vi "Async Thread.vi"(11 "TCP网络连接引用句柄":refnum<k5>) -> ()   [LabVIEW 2019, in "HTTP Server.lvlib"]
uses:
  HTTP Server.lvlib
  Async Thread.ctl
panel:
  out "路径":path
  in  "停止":bool
  out "添加的路径":path
  out "error out":errorcluster caption="错误输出"
  in  "error in (no error)":errorcluster caption="错误输入（无错误）"
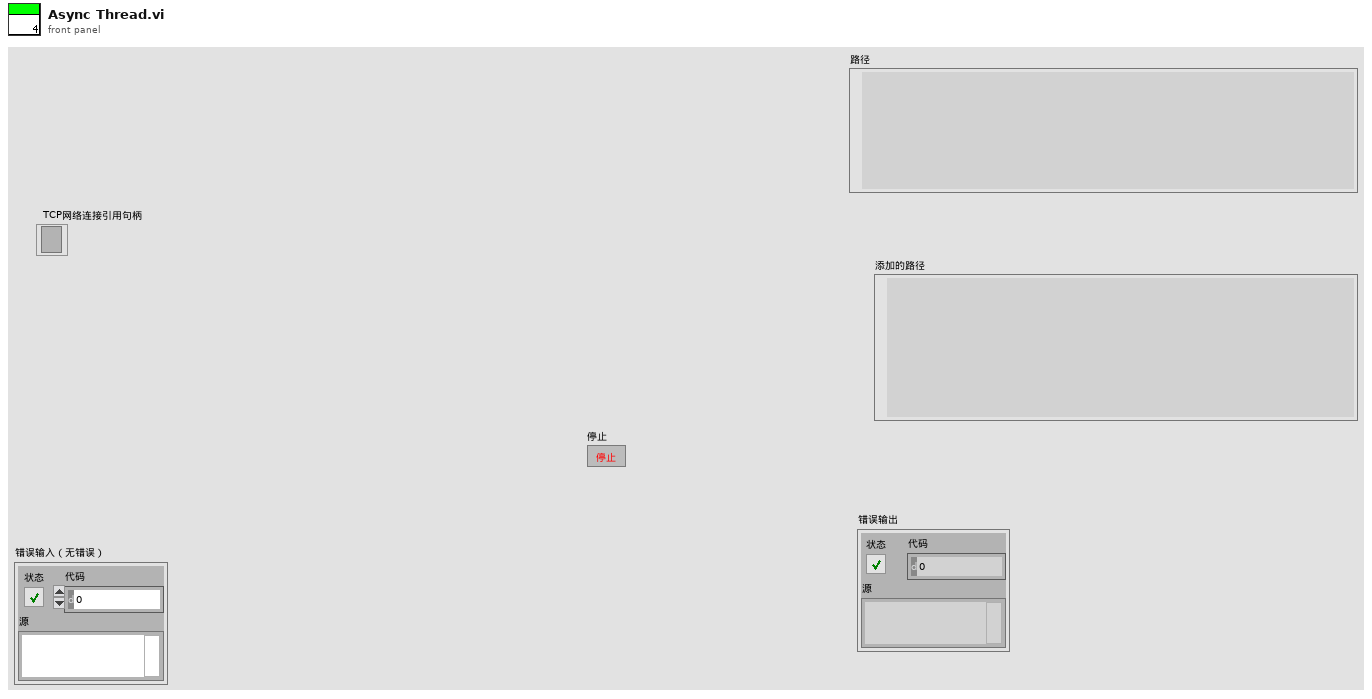
[diagram p1: front panel]
types:
  T1 = typedef "HTTP Server.lvlib/Async Thread.ctl" = cluster{"HTTP报文":string, "请求报文首部":cluster{"请求行":cluster{"方法":string, "URI":string, "表单数据":cluster{"key":string[], "value":string[]}, "HTTP版本":string}, "首部字段":cluster{"key":string[], "value":string[]}}, "请求报文主体":string, "响应报文主体":string, "响应代码":u16, "响应报文首部":string, "Redis TCP引用":refnum<k5>}
  T2 = enum32{"invalid app kind", "Development System", "Run Time System", "Student Edition", "Embedded LabVIEW", "Evaluation", "Custom"}
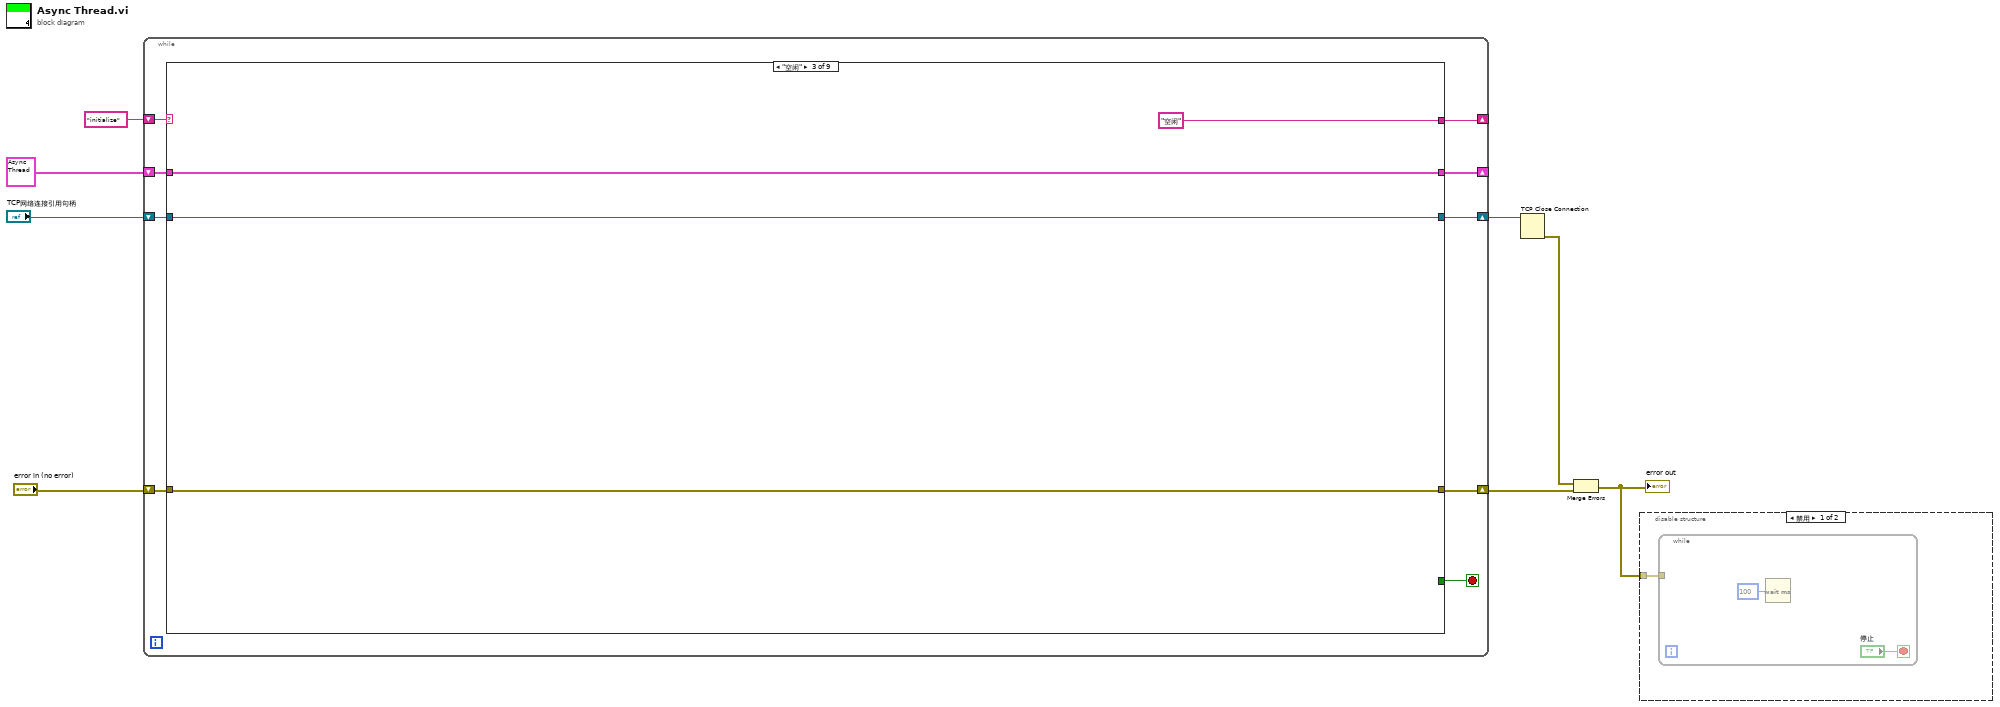
[diagram p0: block diagram]
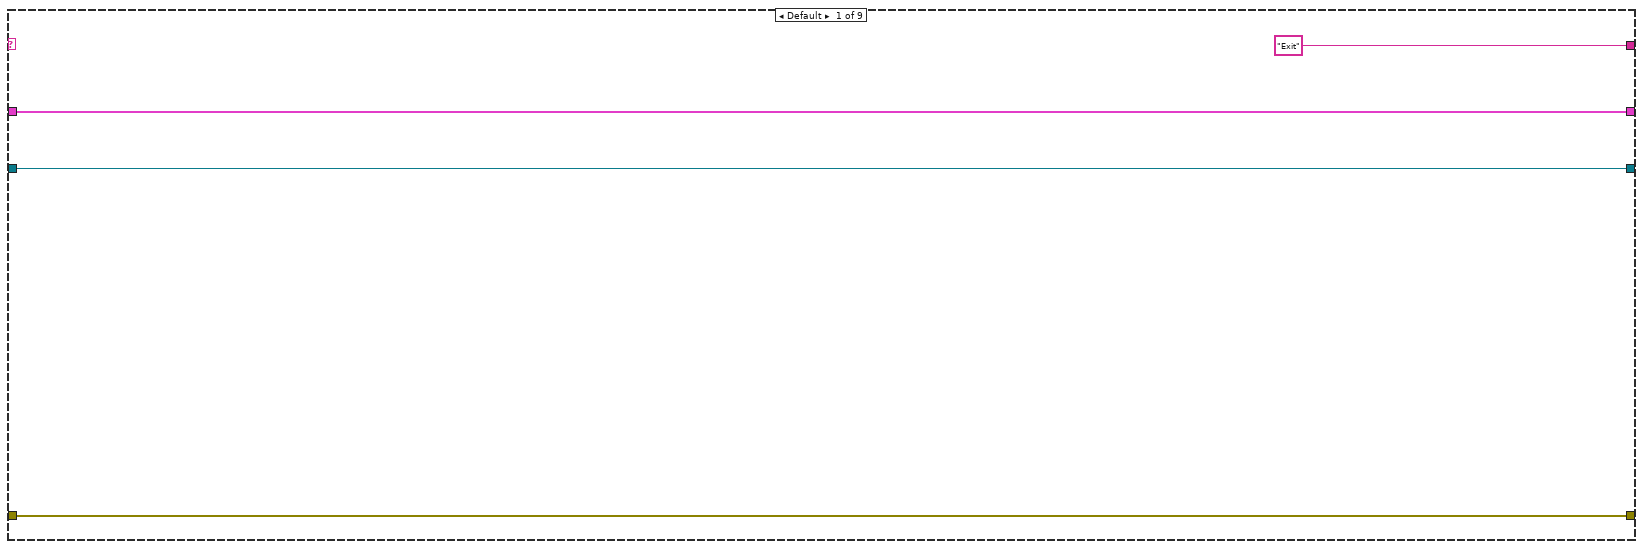
[diagram p3: hidden frame]
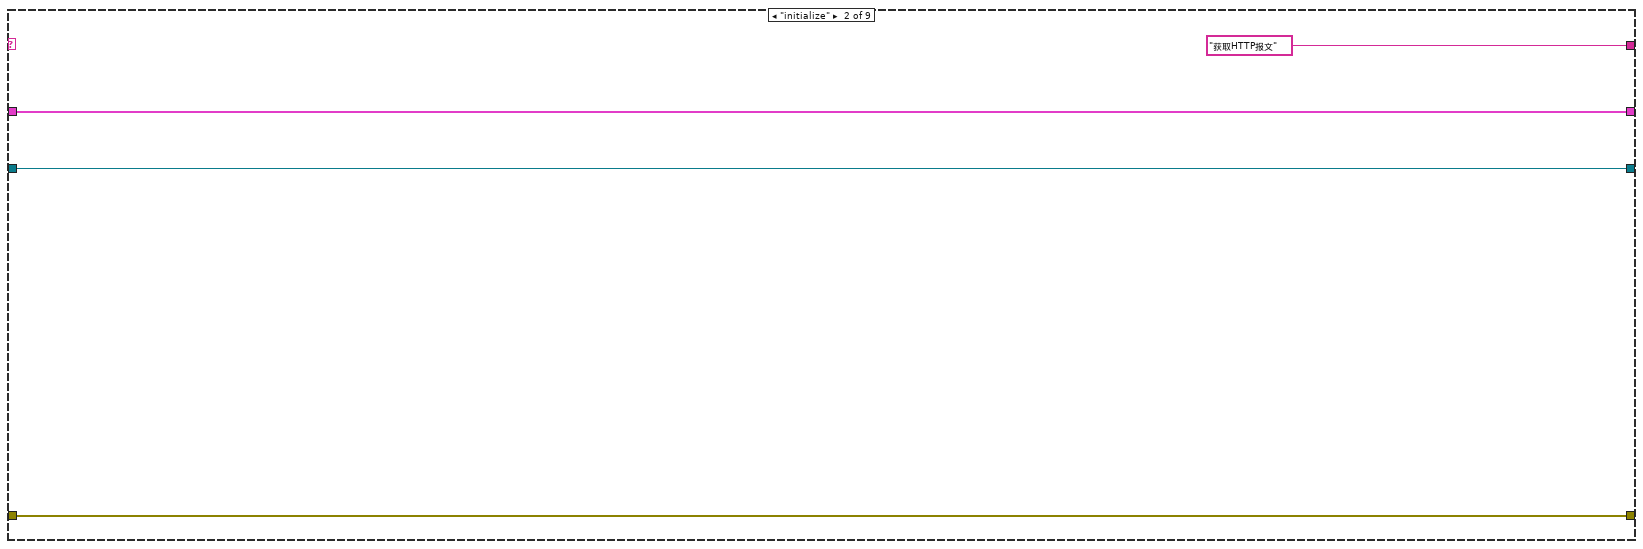
[diagram p4: hidden frame]
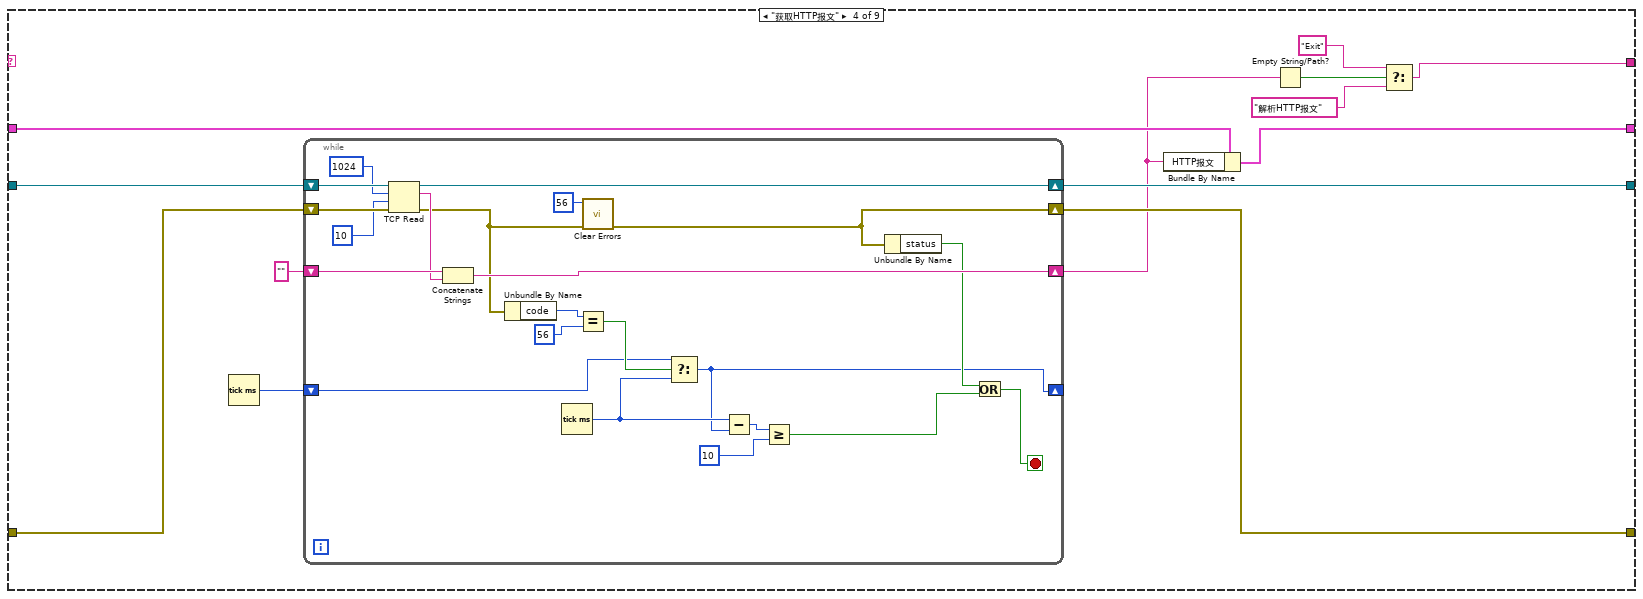
[diagram p5: hidden frame]
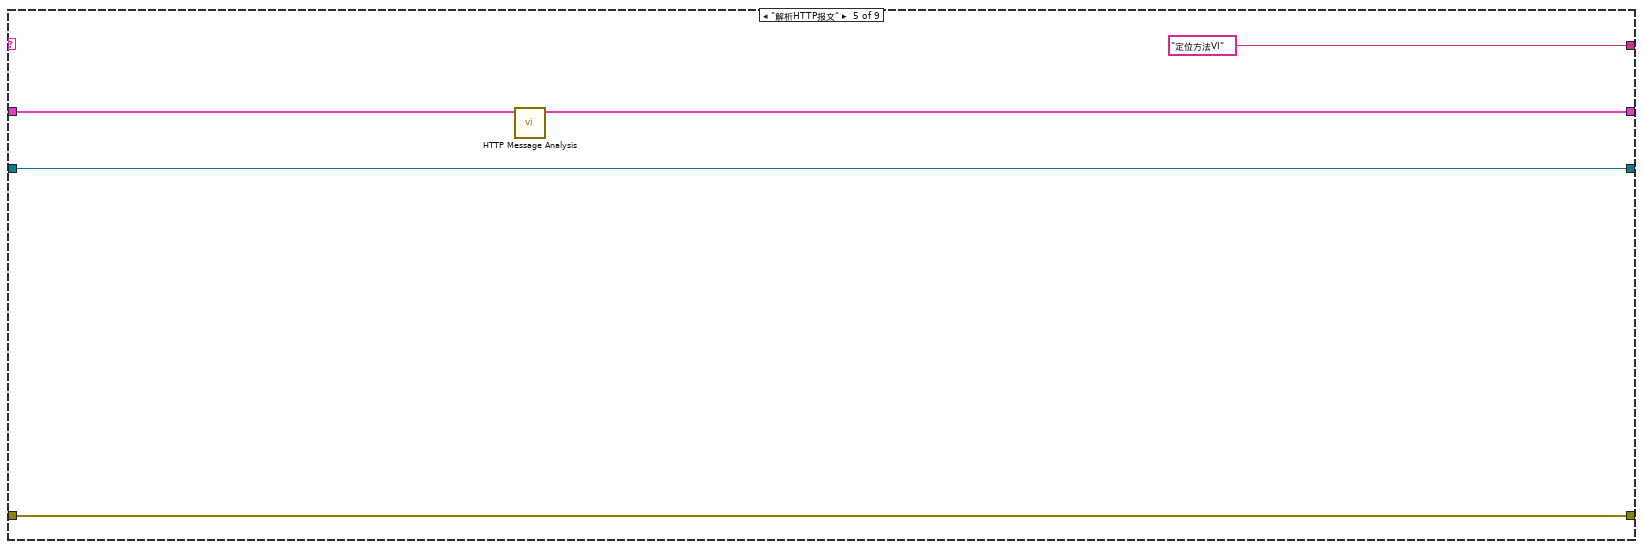
[diagram p6: hidden frame]
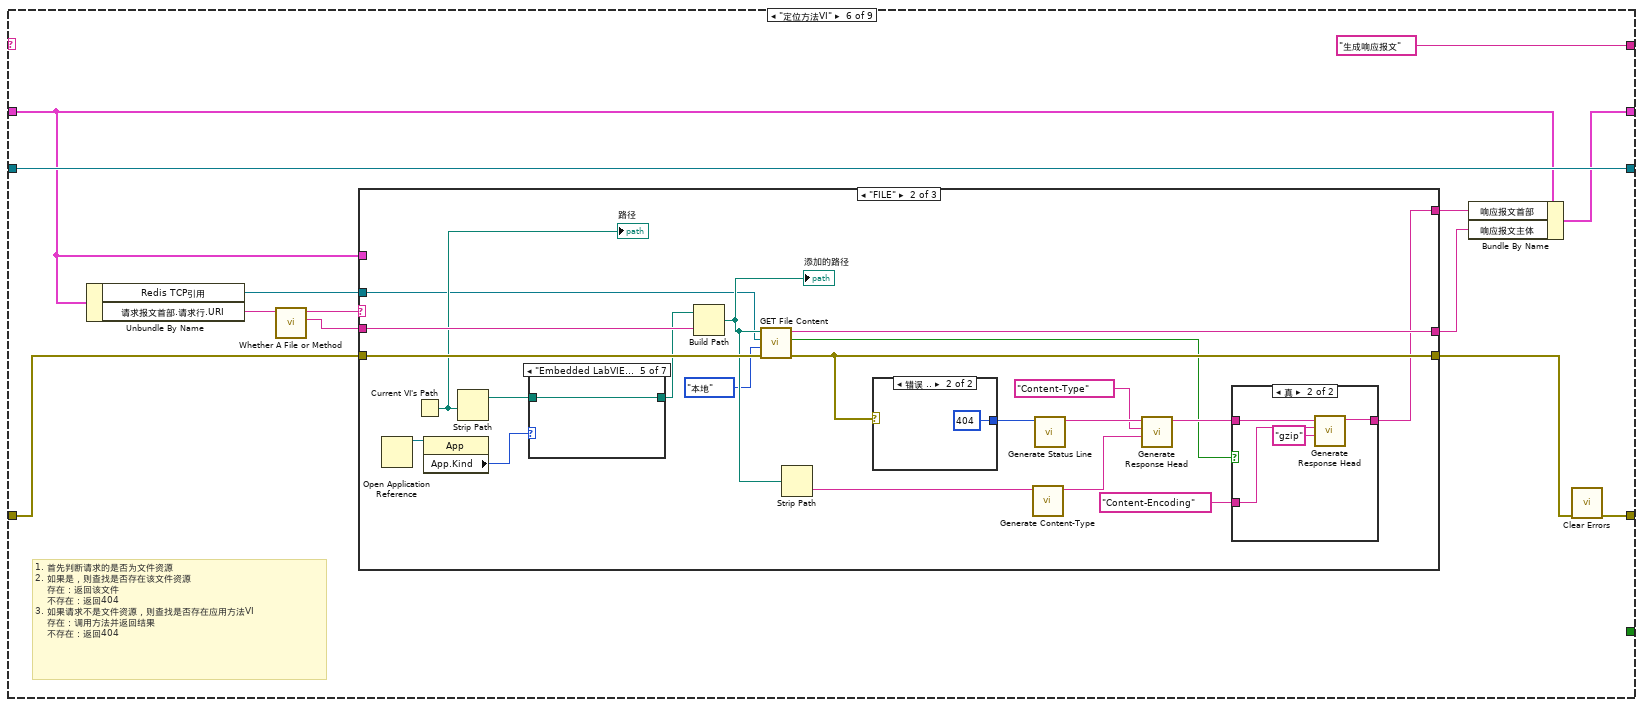
[diagram p7: hidden frame]
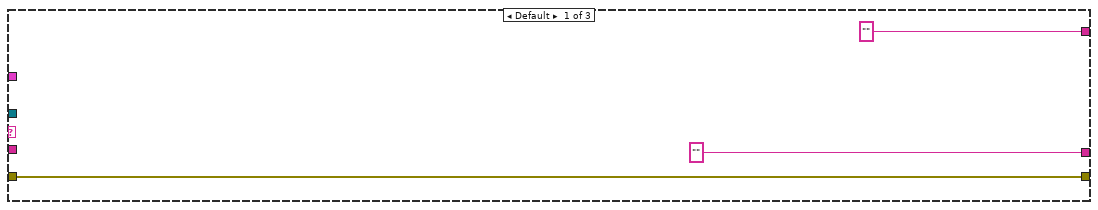
[diagram p8: hidden frame]
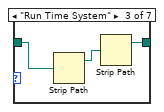
[diagram p12: hidden frame]
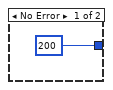
[diagram p16: hidden frame]
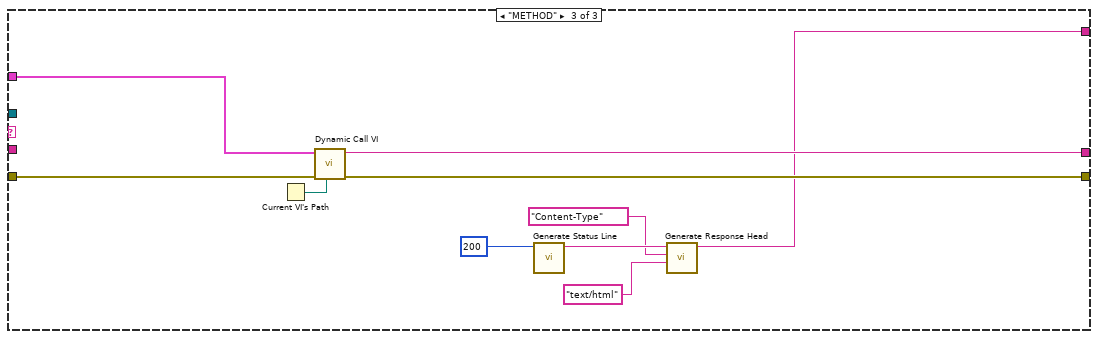
[diagram p17: hidden frame]
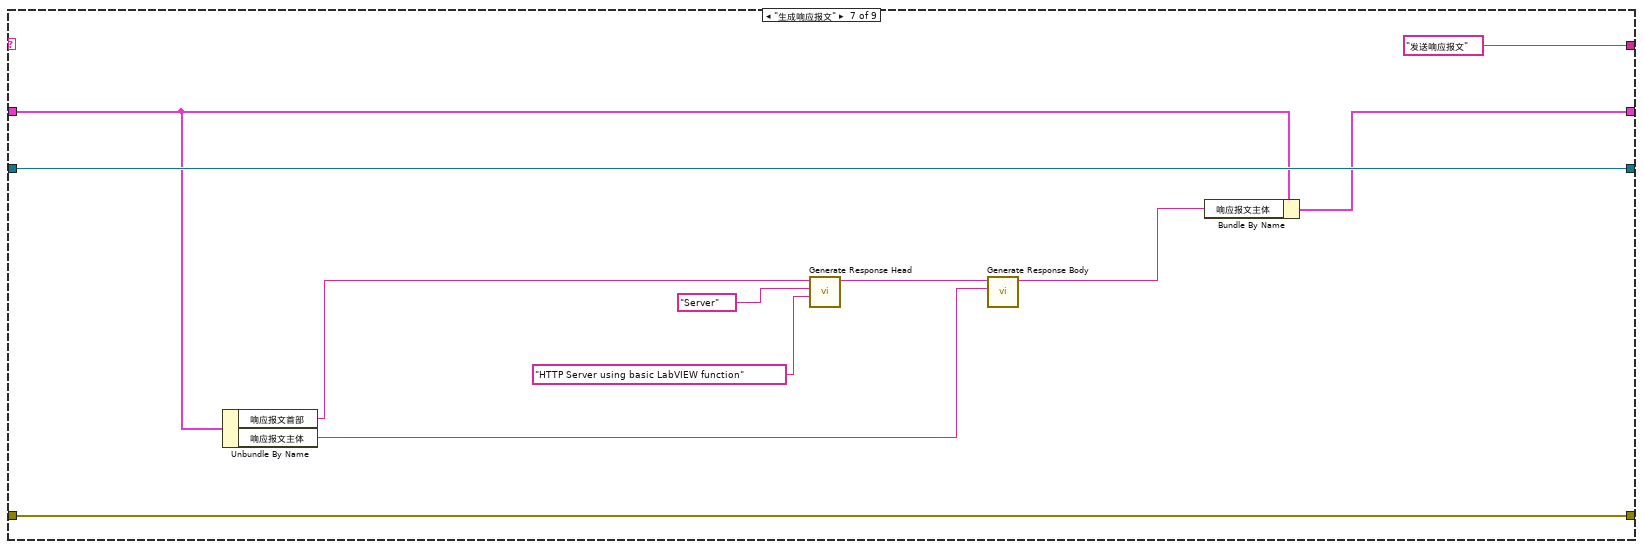
[diagram p18: hidden frame]
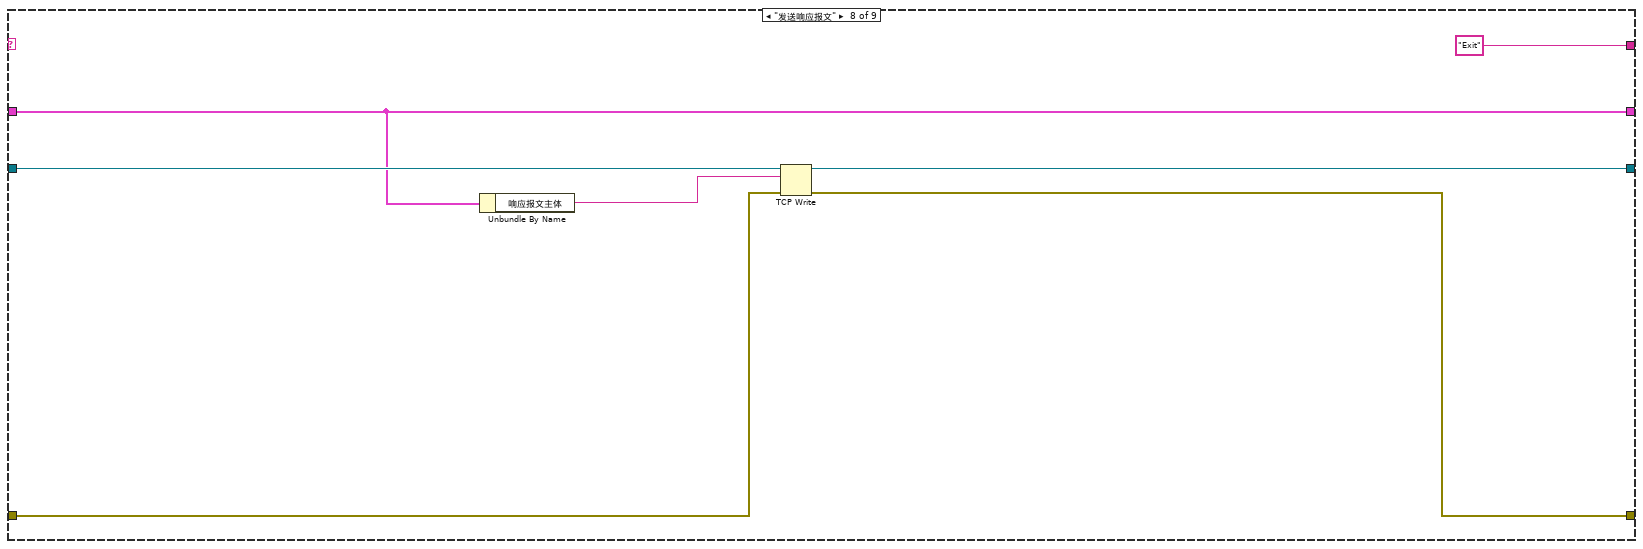
[diagram p19: hidden frame]
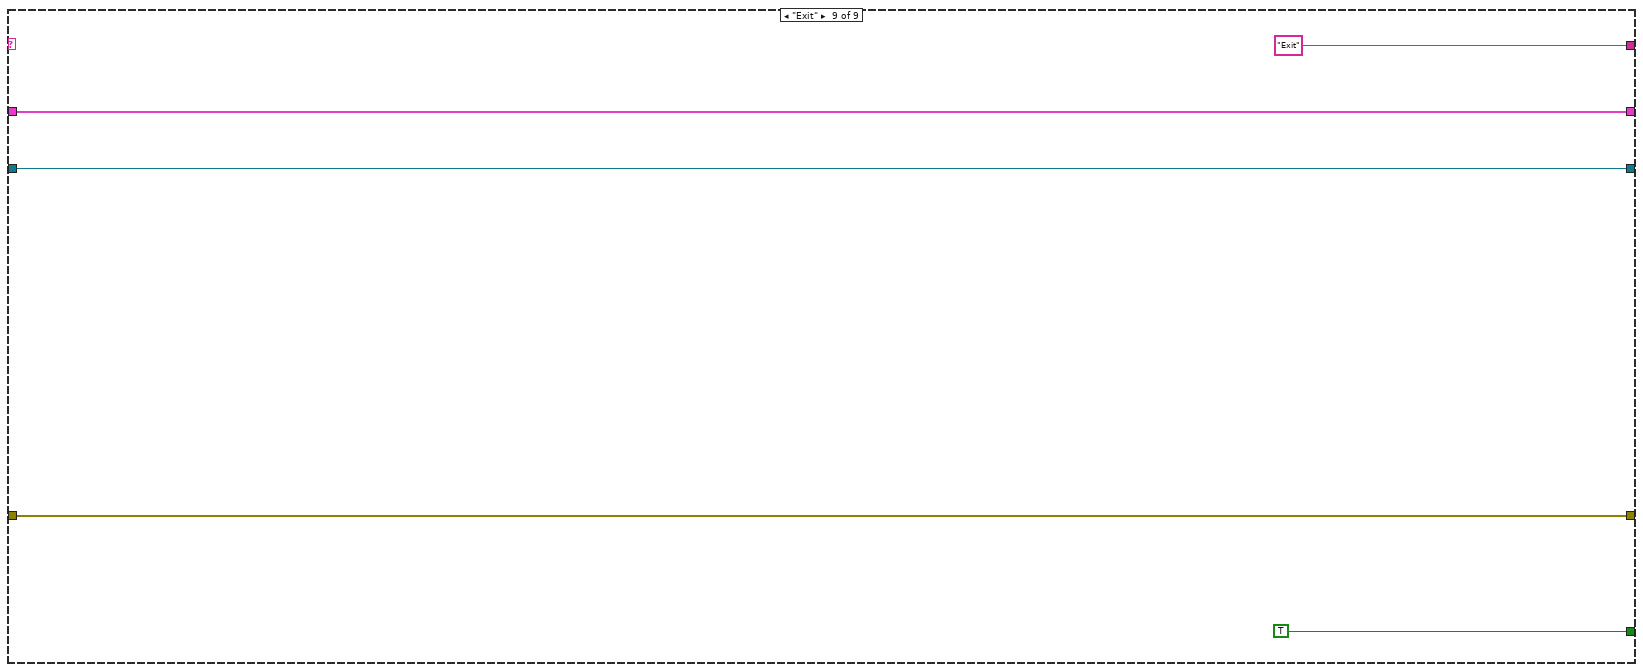
[diagram p20: hidden frame]
diagram:
  n1 = while {
    shift-right: [w12] -> _
    shift-left: "initialize" -> [w17]
    shift-right: [w11] -> w4
    shift-left: "TCP网络连接引用句柄" -> [w15]
    shift-right: [w13] -> w2
    shift-left: "error in (no error)" -> [w14]
    shift-right: [w9] -> _
    shift-left: T1 {"HTTP报文"="", "请求报文首部"={"请求行"={"方法"="", "URI"="", "表单数据"={"key"=[], "value"=[]}, "HTTP版本"=""}, "首部字段"={"key"=[], "value"=[]}}, "请求报文主体"="", "响应报文主体"="", "响应代码"=0, "响应报文首部"="", "Redis TCP引用"=refnum} ("簇") -> [w10]
    stop <- w16 stop-if-true
    n2 = case shown="\"空闲\"" w17 {
      tunnel: [_ _ _ _ _ _ _ _ TRUE] -> w16
      tunnel: w15 -> [w21 w24 w28 w42 w68 w80 w142 w149 w154]
      tunnel: w14 -> [w20 w23 w29 w40 w69 w81 w143 w147 w153]
      tunnel: [w20 w23 w29 w39 w69 w72 w143 w146 w153] -> w13
      tunnel: ["Exit" "获取HTTP报文" "空闲" w30 "定位方法VI" "生成响应报文" "发送响应报文" "Exit" "Exit"] -> w12
      tunnel: [w21 w24 w28 w41 w68 w80 w142 w148 w154] -> w11
      tunnel: w10 -> [w19 w22 w27 w38 w66 w75 w139 w145 w151]
      tunnel: [w19 w22 w27 w37 w65 w79 w140 w145 w151] -> w9
      frame Default {
      }
      frame "initialize" {
      }
      frame "空闲" {
      }
      frame "获取HTTP报文" {
        n3 = Tick Count (ms)() -> (millisecond timer value=w35:u32)
        n4 = while {
          shift-right: [w63] -> w41
          shift-left: w42 -> [w64]
          shift-right: [w55] -> w39
          shift-left: w40 -> [w62]
          shift-right: [w57] -> w34
          shift-left: "" -> [w59]
          shift-right: [w46] -> _
          shift-left: w35 -> [w48]
          stop <- w53 stop-if-true
          n5 = TCP Read(connection ID=w64, bytes to read=1024 ("读取的字节"), error in (no error)=w62, 9:10 ("超时毫秒(25000)")) -> (connection ID out=w63:refnum<k5>, data out=w58:string, error out=w52:errorcluster)  [unwired: 1 in]
          n6 = Concatenate Strings(w59, w58) -> (w57:string)
          n7 = Unbundle By Name(w52) -> ("code"=w51:i32)
          n8 = Tick Count (ms)() -> (millisecond timer value=w47:u32)
          n9 = Equal?(x=w51, y=56) -> (x = y?=w49:bool)
          n10 = call <vilib>:"Clear Errors.vi"("error in (no error)"=w52, "specific error code to clear (0: all)"=56) -> ("error out"=w55:errorcluster)  [unwired: 4 in, 1 out]
          n11 = Select(t=w48, s=w49, f=w47) -> (s? t:f=w46:u32)
          n12 = Subtract(x=w47, y=w46) -> (x-y=w45:u32)
          n13 = Greater Or Equal?(x=w45, y=u32 10) -> (x >= y?=w43:bool)
          n14 = Unbundle By Name(w55) -> ("status"=w54:bool)
          n15 = Or(x=w54, y=w43) -> (x .or. y?=w53:bool)
        }
        n16 = Bundle By Name(cluster=w38, "HTTP报文"=w34) -> (w37:T1)
        n17 = Empty String/Path?(string/path=w34) -> (empty?=w33:bool)
        n18 = Select(t="Exit", s=w33, f="解析HTTP报文") -> (s? t:f=w30:string)
      }
      frame "解析HTTP报文" {
        n19 = call "HTTP Message Analysis.vi"("异步调用线程簇输入"=w66) -> ("异步调用线程簇输出"=w65:T1)  [unwired: 10 in]
      }
      frame "定位方法VI" {
        # "1. 首先判断请求的是否为文件资源\n2. 如果是，则查找是否存在该文件资源\n    存在：返回该文件\n    不存在：返回404\n3. 如果请求不是文件资源，则查找是否存在应用方法VI\n    存在：调用方法并返回结果\n    不存在：返回404"
        n20 = Unbundle By Name(w75) -> ("Redis TCP引用"=w70:refnum<k5>, "请求报文首部.请求行.URI"=w77:string)
        n21 = call "Whether A File or Method.vi"("URI"=w77) -> ("Path(Win)"=w74:string, "Type"=w76:string)  [unwired: 9 in]
        n22 = case shown="\"FILE\"" w76 {
          tunnel: w81 -> [w85 w105 w132]
          tunnel: [w85 w103 w131] -> w73
          tunnel: ["" ("响应报文主体") w104 w130] -> w78
          tunnel: w75 -> [_ _ w128]
          tunnel: w74 -> [_ w106 _]
          tunnel: ["" ("HEADOUT") w87 w125] -> w71
          tunnel: w70 -> [_ w91 _]
          frame Default {
          }
          frame "FILE" {
            n23 = Open Application Reference() -> (3:w94:refnum<vi>)  [unwired: 4 in, 1 out]
            n24 = Current VI's Path() -> (path=w93:path)
            "路径" <- w93
            n25 = property class="App"(reference=w94) -> ("App.Kind"=w95:T2)  [unwired: 1 in, 2 out]
            n26 = Strip Path(path=w93) -> (stripped path=w96:path)  [unwired: 1 out]
            n27 = case shown="\"Embedded LabVIEW\"" w95 {
              tunnel: w96 -> [w112 w113 w115 w117 w118 w119 w120]
              tunnel: [w112 w113 w116 w117 w118 w119 w120] -> w92
              frame "invalid app kind", Default {
              }
              frame "Development System" {
              }
              frame "Run Time System" {
                n28 = Strip Path(path=w115) -> (stripped path=w114:path)  [unwired: 1 out]
                n29 = Strip Path(path=w114) -> (stripped path=w116:path)  [unwired: 1 out]
              }
              frame "Student Edition" {
              }
              frame "Embedded LabVIEW" {
              }
              frame "Evaluation" {
              }
              frame "Custom" {
              }
            }
            n30 = Build Path(base path=w92, name or relative path=w106) -> (appended path=w101:path)
            "添加的路径" <- w101
            n31 = call "GET File Content.vi"("错误输入"=w105, "文件源"=enum16{"本地", "Redis"}."本地", "Redis TCP引用"=w91, "File Path"=w101) -> ("错误输出"=w103:errorcluster, "gzip"=w88:bool, "File Content"=w104:string)  [unwired: 5 in]
            n32 = Strip Path(path=w101) -> (name=w100:string)  [unwired: 1 out]
            n33 = case shown="错误 .." w103 {
              tunnel: [u16 200 u16 404] -> w102
              frame No Error {
              }
              frame Error {
              }
            }
            n34 = call "Generate Content-Type.vi"("Filename"=w100) -> ("Content-Type"=w97:string)  [unwired: 10 in]
            n35 = call "Generate Status Line.vi"("状态码"=w102) -> ("状态行"=w99:string)  [unwired: 10 in]
            n36 = call "Generate Response Head.vi"("Value"=w97, "Header"="Content-Type", "HEADIN"=w99) -> ("HEADOUT"=w89:string)  [unwired: 8 in]
            n37 = case shown="真" w88 {
              tunnel: w89 -> [w107 w111]
              tunnel: [w107 w110] -> w87
              tunnel: "Content-Encoding" -> [_ w109]
              frame False {
              }
              frame True {
                n38 = call "Generate Response Head.vi"("Value"="gzip", "Header"=w109, "HEADIN"=w111) -> ("HEADOUT"=w110:string)  [unwired: 8 in]
              }
            }
          }
          frame "METHOD" {
            n39 = Current VI's Path() -> (path=w129:path)
            n40 = call "Dynamic Call VI.vi"("VI路径"=w129, "错误输入（无错误）"=w132, "异步调用线程簇"=w128) -> ("错误输出"=w131:errorcluster, "响应报文主体"=w130:string)  [unwired: 7 in]
            n41 = call "Generate Status Line.vi"("状态码"=u16 200) -> ("状态行"=w126:string)  [unwired: 10 in]
            n42 = call "Generate Response Head.vi"("Value"="text/html", "Header"="Content-Type", "HEADIN"=w126) -> ("HEADOUT"=w125:string)  [unwired: 8 in]
          }
        }
        n43 = Bundle By Name(cluster=w75, "响应报文首部"=w71, "响应报文主体"=w78) -> (w79:T1)
        n44 = call <vilib>:"Clear Errors.vi"("error in (no error)"=w73) -> ("error out"=w72:errorcluster)  [unwired: 5 in, 1 out]
      }
      frame "生成响应报文" {
        n45 = Unbundle By Name(w139) -> ("响应报文首部"=w133:string, "响应报文主体"=w138:string)
        n46 = call "Generate Response Head.vi"("Value"="HTTP Server using basic LabVIEW function", "Header"="Server", "HEADIN"=w133) -> ("HEADOUT"=w136:string)  [unwired: 8 in]
        n47 = call "Generate Response Body.vi"("Body"=w138, "HEADIN"=w136) -> ("MessageOUT"=w137:string)  [unwired: 9 in]
        n48 = Bundle By Name(cluster=w139, "响应报文主体"=w137) -> (w140:T1)
      }
      frame "发送响应报文" {
        n49 = Unbundle By Name(w145) -> ("响应报文主体"=w144:string)
        n50 = TCP Write(connection ID=w149, data in=w144, error in (no error)=w147) -> (connection ID out=w148:refnum<k5>, error out=w146:errorcluster)  [unwired: 1 in, 1 out]
      }
      frame "Exit" {
      }
    }
  }
  n51 = TCP Close Connection(connection ID=w4) -> (error out=w3:errorcluster)  [unwired: 2 in, 1 out]
  n52 = Merge Errors(w3, w2) -> (w1:errorcluster)
  "error out" <- w1
  n53 = disable-structure shown="禁用" {
    disable-tunnel: w1 -> [w156 _]
    frame Disabled {
      n54 = while {
        tunnel: w156 -> [_]
        stop <- "停止" stop-if-true
        n55 = Wait (ms)(milliseconds to wait=u32 100 ("等待时间（毫秒）")) -> ()  [unwired: 1 out]
      }
    }
    frame Enabled {
    }
  }
